vi "Read Rate Interval (s).vi"(8 "error in (no error)":errorcluster, 11 "AInterestAccount in":refnum<class "AInterestAccount.lvclass">) -> (0 "error out":errorcluster, 2 "Rate Interval (s)":u32, 3 "AInterestAccount out":refnum<class "AInterestAccount.lvclass">)   [LabVIEW 2020, in "AInterestAccount.lvclass"]
uses:
  AInterestAccount.lvclass
  AInterestAccount.lvclass/AInterestAccount.ctl
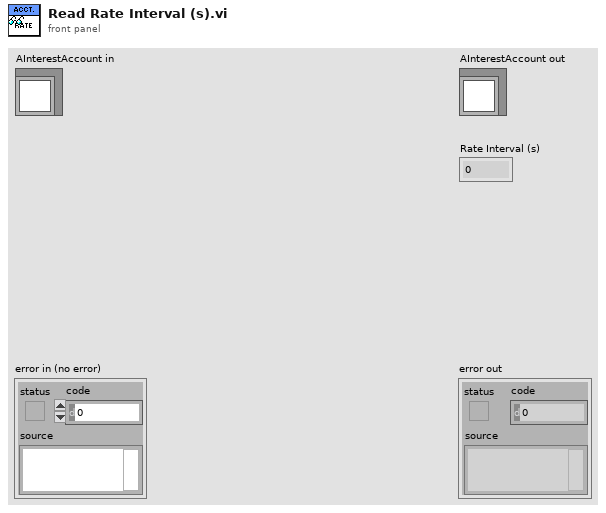
[diagram p1: front panel]
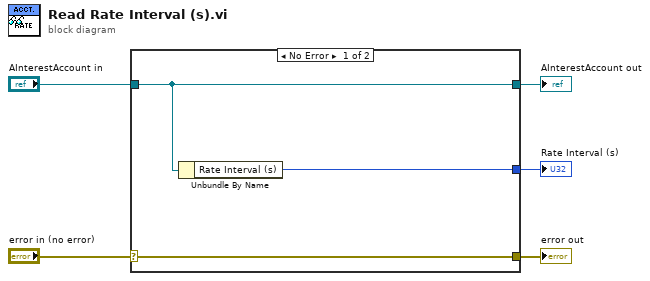
[diagram p0: block diagram]
diagram:
  n1 = case shown="No Error" "error in (no error)" {
    selector: "error in (no error)" -> [w8 w9]
    tunnel: [w8 w9] -> w4
    tunnel: [w7 w10] -> w2
    tunnel: "AInterestAccount in" -> [w7 w10]
    tunnel: [w6 _] -> w1
    frame No Error {
      n2 = Unbundle By Name(w7) -> ("Rate Interval (s)"=w6:u32)
    }
    frame Error {
    }
  }
  "error out" <- w4
  "AInterestAccount out" <- w2
  "Rate Interval (s)" <- w1
